vi "ep_FFT Spectrum.vi"(8 "error in (no error)":errorcluster, 10 "# of bins":i32, 11 "resampled signal":dbl[](array[numeric])) -> (0 "error out":errorcluster, 2 "phase":dbl[](array[numeric]), 3 "magnitude":dbl[](array[numeric]))   [LabVIEW 2013, in "NI_EP_Power Measurement.lvlib"]
uses:
  <vilib>/addons/Electrical Power/Power Measurement/NI_EP_Power Measurement.lvlib
  <vilib>/Analysis/NI_AALPro.lvlib
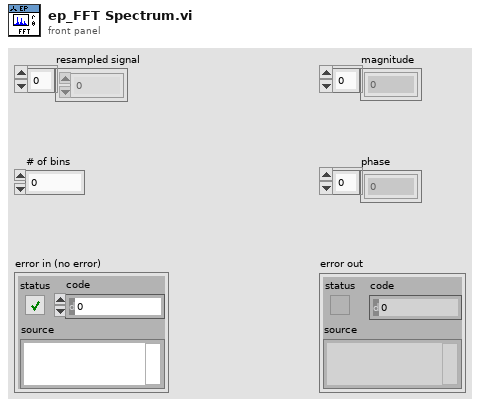
[diagram p1: front panel]
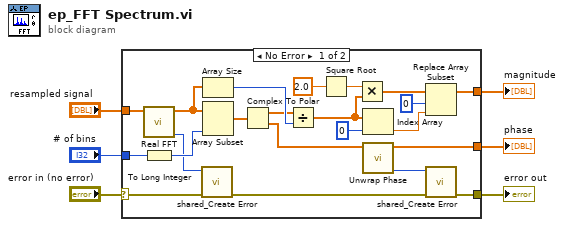
[diagram p0: block diagram]
diagram:
  n1 = case shown="No Error" "error in (no error)" {
    selector: "error in (no error)" -> [w12 w29]
    tunnel: "resampled signal" -> [w11 _]
    tunnel: [w10 _] -> w4
    tunnel: [w9 _] -> w3
    tunnel: [w8 w29] -> w2
    tunnel: "# of bins" -> [w7 _]
    frame No Error {
      n2 = call <vilib>:"Real FFT.vi"("X"=w11) -> ("error"=w13:i32, "FFT {X}"=w24:cdb[])  [unwired: 9 in]
      n3 = To Long Integer(number=w7) -> (32bit integer=w14:i32)
      n4 = call <vilib>:"shared_Create Error.vi"("error in (no error)"=w12, "error code (0)"=w13) -> ("error out"=w27:errorcluster)  [unwired: 9 in]
      n5 = Array Size(array=w24) -> (size(s)=w25:i32)
      n6 = Array Subset(array=w24, length=w14) -> (w22:cdb[])  [unwired: 1 in]
      n7 = Complex To Polar(r * e^(i*theta)=w22) -> (r=w23:dbl[], theta=w26:dbl[])
      n8 = Divide(x=w23, y=w25) -> (x/y=w16:dbl[])
      n9 = Square Root(x=2.0) -> (sqrt(x)=w17:dbl)
      n10 = Multiply(x=w17, y=w16) -> (x*y=w18:dbl[])
      n11 = Index Array(array=w16, index=0) -> (element=w15:dbl)
      n12 = call <vilib>:"Unwrap Phase.vi"("Phase"=w26) -> ("error"=w28:i32, "Unwrapped Phase"=w9:dbl[])  [unwired: 9 in]
      n13 = Replace Array Subset(array=w18, new element=w15, index=0) -> (w10:dbl[])
      n14 = call <vilib>:"shared_Create Error.vi"("error in (no error)"=w27, "error code (0)"=w28) -> ("error out"=w8:errorcluster)  [unwired: 9 in]
    }
    frame Error {
    }
  }
  "error out" <- w2
  "magnitude" <- w4
  "phase" <- w3
